vi "pmu_Read Time.vi"(8 "error in (no error)":errorcluster, 11 "system info in":refnum<class "PMU System Info.lvclass">) -> (0 "error out":errorcluster, 1 "time quality":u8, 2 "time stamp":timestamp, 3 "system info out":refnum<class "PMU System Info.lvclass">)   [LabVIEW 2011, in "NI_EP_PMU.lvlib" / "PMU System Info.lvclass"]
uses:
  <vilib>/addons/Electrical Power/PMU/Common/Classes/PMU System Info/PMU System Info.lvclass
  <vilib>/addons/Electrical Power/PMU/Common/Classes/PMU System Info/PMU System Info.lvclass/PMU System Info.ctl
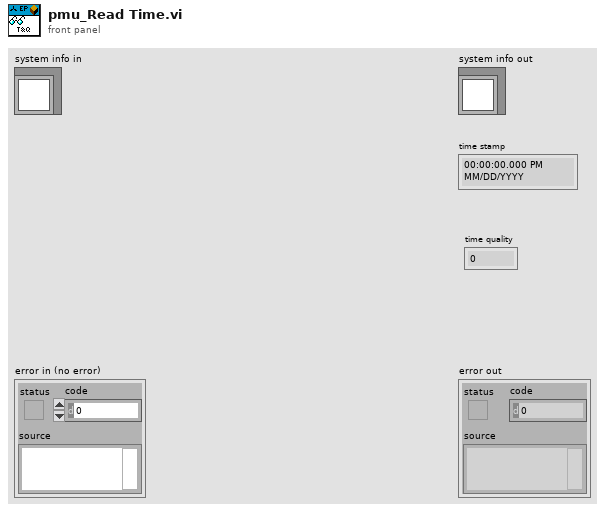
[diagram p1: front panel]
types:
  T1 = typedef "NI_EP_PMU.lvlib/pmu_Time&Quality.ctl" = cluster{"time stamp":timestamp, "time quality":u8}
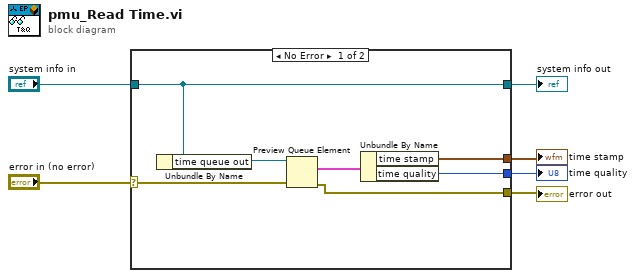
[diagram p0: block diagram]
diagram:
  n1 = case shown="No Error" "error in (no error)" {
    selector: "error in (no error)" -> [w8 w14]
    tunnel: [w13 w15] -> w4
    tunnel: "system info in" -> [w13 w15]
    tunnel: [w12 _] -> w3
    tunnel: [w11 _] -> w2
    tunnel: [w7 w14] -> w1
    frame No Error {
      n2 = Unbundle By Name(w13) -> ("time queue out"=w10:refnum<queue>)
      n3 = Preview Queue Element(queue=w10, error in (no error)=w8) -> (element=w9:T1, error out=w7:errorcluster)  [unwired: 1 in, 2 out]
      n4 = Unbundle By Name(w9) -> ("time stamp"=w12:timestamp, "time quality"=w11:u8)
    }
    frame Error {
    }
  }
  "error out" <- w1
  "system info out" <- w4
  "time stamp" <- w3
  "time quality" <- w2
